vi "FuncImg-Set window state.vi"(8 "error in (no error)":errorcluster, 11 "Front Panel Window:State":T1(ring)=enum."Maximized") -> (0 "error out":errorcluster)   [LabVIEW 2013]
uses:
  Global variables/gl_Functional Imaging-Global variables.vi
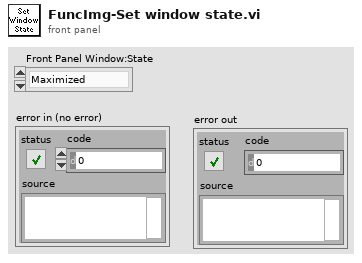
[diagram p1: front panel]
types:
  T1 = enum32{"Invalid", "Standard", "Closed", "Hidden", "Minimized", "Maximized"}
  T2 = typedef "Functional Imging UI Refs.ctl" = cluster{"Menu ref":refnum<k9>, "Image control":refnum<vi>, "VI ref":refnum<vi>, "XGrapher":refnum<vi>, "Smoothing":refnum<vi>, "POI Averaging":refnum<vi>, "Normalize":refnum<vi>, "POI data points in each trial":refnum<vi>, "Channel":refnum<vi>, "Experiment data folder path":refnum<vi>, "[ROI vis]":refnum<vi>, "[Groups] visbl":T3, "Group Name":refnum<vi>, "POI index":refnum<vi>, "Trial No.":refnum<vi>, "Intensity Zoom":refnum<vi>, "Trial Cursor Enabled":refnum<vi>, "Number of Trials (ind 1)":refnum<vi>, "Number of Trials (ind 2)":refnum<vi>, "MiniScans Available":refnum<vi>, "POI Available":refnum<vi>, "Defer graph updates":refnum<vi>, "Waveform selector":refnum<vi>, "#of selected POI":refnum<vi>, "#of selected MiniScans":refnum<vi>, "#of selected groups":refnum<vi>, "Max Z-Projection":refnum<vi>, "Z-Plane Selector":refnum<vi>, "Index of miniscan point to visualise":refnum<vi>, "ROI vis. mode":refnum<vi>, "Total # of points":refnum<vi>, "Index of group clicked on":refnum<vi>, "Pane 1":refnum<vi>, "Pane 2":refnum<vi>, "Pane 3":refnum<vi>, "Pane 4":refnum<vi>, "Pane 5":refnum<vi>, "Pane 6":refnum<vi>, "Deselect all ROI":refnum<vi>, "Deselect all groups":refnum<vi>}
  T3 = typedef "Groups array referecne.ctl" = refnum<vi>
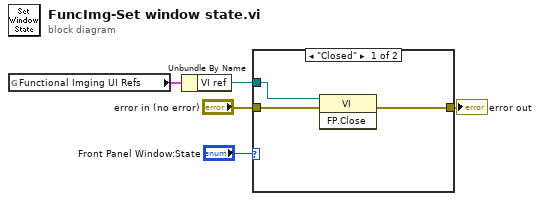
[diagram p0: block diagram]
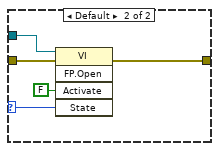
[diagram p2: hidden frame]
diagram:
  n1 = global read "gl_Functional Imaging-Global variables.vi" "Functional Imging UI Refs"() -> (w4:T2)
  n2 = Unbundle By Name(w4) -> ("VI ref"=w5:refnum<vi>)
  n3 = case shown="\"Closed\"" "Front Panel Window:State" {
    selector: "Front Panel Window:State" -> [_ w10]
    tunnel: "error in (no error)" -> [w6 w12]
    tunnel: [w8 w11] -> w2
    tunnel: w5 -> [w7 w9]
    frame "Closed" {
      n4 = invoke class="VI" method="FP.Close"(reference=w7, error in=w6) -> (error out=w8:errorcluster)  [unwired: 1 in, 2 out]
    }
    frame Default {
      n5 = invoke class="VI" method="FP.Open"(reference=w9, error in=w12, "Activate"=FALSE ("Activate?"), "State"=w10) -> (error out=w11:errorcluster)  [unwired: 1 in, 4 out]
    }
  }
  "error out" <- w2
